vi "加标回收数据组合 (子VI).vi"(9 "小时数据发送次数":i32, 10 "数据":string[][](array[string]), 11 "污染物编码":string) -> (2 "组合输出":string, 3 "datatime":string)   [LabVIEW 2016, in "数据传输系统-05.lvlib"]
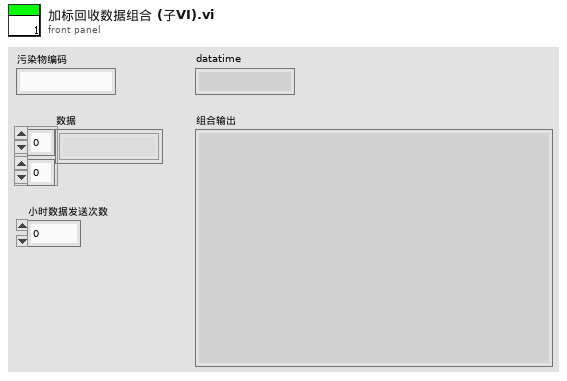
[diagram p1: front panel]
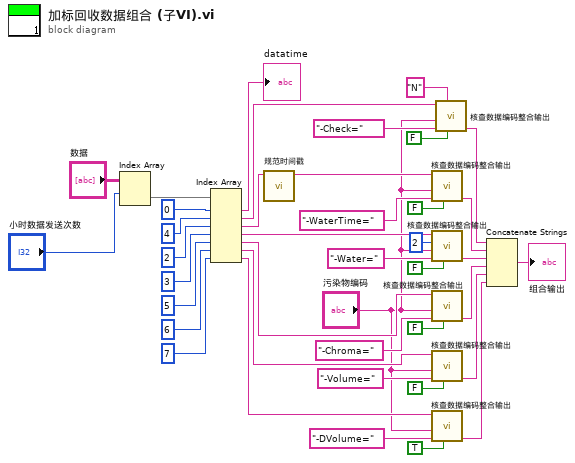
[diagram p0: block diagram]
diagram:
  n1 = Index Array(array="数据", index (row)="小时数据发送次数") -> (element=w4:string[])  [unwired: 1 in]
  n2 = Index Array(array=w4, index #1=0 ("索引"), index #2=4 ("索引"), index #3=2 ("索引"), index #4=3 ("索引"), index #5=5 ("索引"), index #6=6 ("索引"), index #7=7 ("索引")) -> (element #1=→"datatime":string, element #2=w10:string, element #3=w39:string, element #4=w16:string, element #5=w18:string, element #6=w21:string, element #7=w22:string)
  n3 = call "规范时间戳.vi"("字符串"=w39) -> ("result string"=w40:string)  [unwired: 10 in]
  n4 = call "核查数据编码整合输出.vi"("字段结束"=FALSE, "数据类型"="-WaterTime=", "污染物编码"="污染物编码", "数据值"=w40) -> ("编码输出"=w26:string)  [unwired: 7 in]
  n5 = call "核查数据编码整合输出.vi"("字段结束"=FALSE, "数据类型"="-Water=", "污染物编码"="污染物编码", "数据精度"=2, "数据值"=w16) -> ("编码输出"=w27:string)  [unwired: 6 in]
  n6 = call "核查数据编码整合输出.vi"("字段结束"=FALSE, "数据类型"="-Chroma=", "污染物编码"="污染物编码", "数据值"=w18) -> ("编码输出"=w28:string)  [unwired: 7 in]
  n7 = call "核查数据编码整合输出.vi"("字段结束"=FALSE, "数据类型"="-Volume=", "污染物编码"="污染物编码", "数据值"=w21) -> ("编码输出"=w29:string)  [unwired: 7 in]
  n8 = call "核查数据编码整合输出.vi"("字段结束"=TRUE, "数据类型"="-DVolume=", "污染物编码"="污染物编码", "数据值"=w22) -> ("编码输出"=w30:string)  [unwired: 7 in]
  n9 = call "核查数据编码整合输出.vi"("字段结束"=FALSE, "数据标识"="N" ("字符串"), "数据类型"="-Check=", "污染物编码"="污染物编码", "数据值"=w10) -> ("编码输出"=w25:string)  [unwired: 6 in]
  n10 = Concatenate Strings(w25, w26, w27, w28, w29, w30) -> (→"组合输出":string)
